vi "Sweeps.vi"   [LabVIEW 2021]
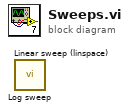
[diagram p0: block diagram]
diagram:
  n1 = call "Log sweep.vi"() -> ()  [unwired: 3 in, 1 out]
  n2 = call "Linear sweep (linspace).vi"() -> ()  [unwired: 3 in, 1 out]
